vi "Find Inherited Test Methods in Test Case.vi"(8 "error in (no error)":errorcluster, 10 "Test Case Class Path":path, 11 "Test Finder In":refnum<class "Test Finder.lvclass">) -> (0 "error out":errorcluster, 2 "Test Methods Out":map{string, path}(c390), 3 "Test Finder Out":refnum<class "Test Finder.lvclass">)   [LabVIEW 2020, in "Test Finder.lvclass"]
uses:
  Test Finder.lvclass
  Test Case/LUnit Test Case.lvclass
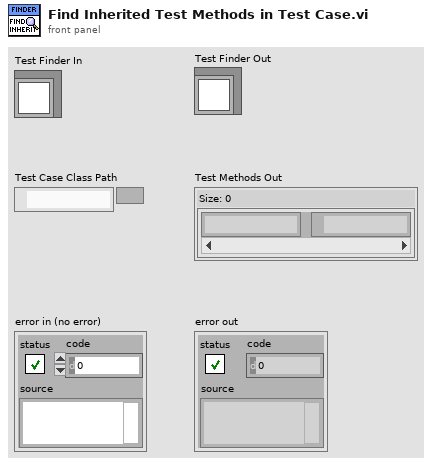
[diagram p1: front panel]
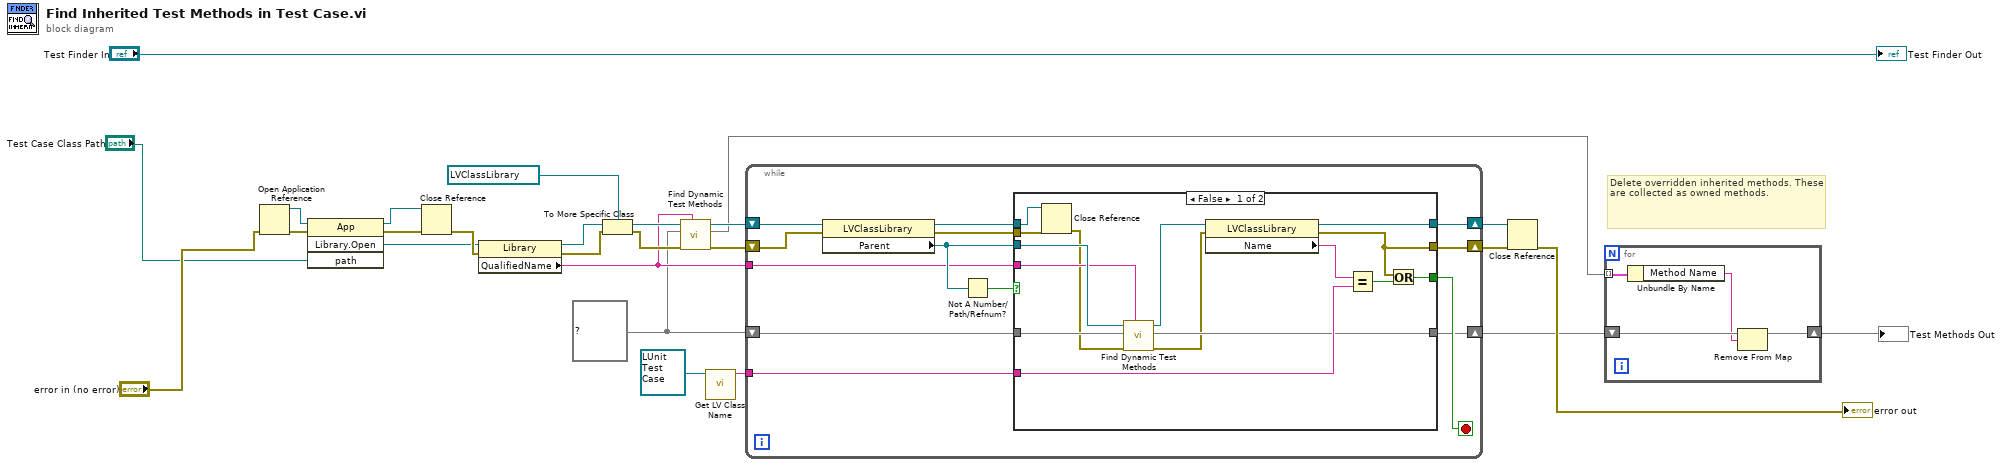
[diagram p0: block diagram]
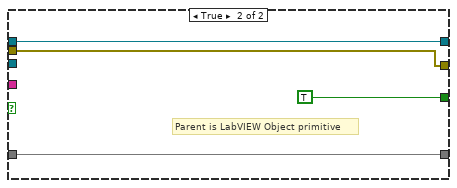
[diagram p2: hidden frame]
diagram:
  w4 = map{string, path} {} ("Test Methods In")
  # "Delete overridden inherited methods. These are collected as owned methods."
  n1 = Open Application Reference(8:"error in (no error)") -> (0:w25:errorcluster, 3:w26:refnum<vi>)  [unwired: 3 in]
  n2 = invoke on="Invoke Node" class="App" method="Library.Open"(reference=w26, error in=w25, "path"="Test Case Class Path") -> (reference out=w23:refnum<vi>, error out=w24:errorcluster, "Open Library"=w10:refnum<vi>)  [unwired: 1 in, 1 out]
  n3 = Close Reference(reference=w23, error in (no error)=w24) -> (error out=w14:errorcluster)
  n4 = property on="Property Node" class="Library"(reference=w10, error in=w14) -> (reference out=w15:refnum<vi>, error out=w13:errorcluster, "QualifiedName"=w5:string)
  n5 = To More Specific Class(target class=refnum<vi> refnum ("Library:Open"), reference=w15, error in=w13) -> (specific class reference=w9:refnum<vi>, error out=w7:errorcluster)
  n6 = call "Find Dynamic Test Methods.vi"("Test Case class name"=w5, "error in (no error)"=w7, "Test Methods In"=w4, "LVClassLibrary in"=w9) -> ("error out"=w6:errorcluster, "Test Methods Out"=w3:map{string, path}, "LVClassLibrary out"=w8:refnum<vi>)  [unwired: 5 in]
  n7 = call <vilib>:"Get LV Class Name.vi"("object"=refnum<class "LUnit Test Case.lvclass"> refnum ("Test Case in")) -> ("class name"=w18:string)  [unwired: 9 in, 1 out]
  n8 = while {
    shift-right: [w28] -> w2
    shift-left: w4 -> [w29]
    shift-right: [w38] -> w19
    shift-left: w8 -> [w31]
    shift-right: [w36] -> w21
    shift-left: w6 -> [w30]
    tunnel: w18 -> [w39]
    tunnel: w5 -> [w27]
    stop <- w37 stop-if-true
    n9 = property on="Property Node" class="LVClassLibrary"(reference=w31, error in=w30) -> (reference out=w33:refnum<vi>, error out=w32:errorcluster, "Parent"=w35:refnum<vi>)
    n10 = Not A Number/Path/Refnum?(number/path/refnum=w35) -> (NaN/Path/Refnum?=w34:bool)
    n11 = case shown="False" w34 {
      tunnel: w39 -> [w54 _]
      tunnel: [w53 w57] -> w38
      tunnel: [w52 TRUE] -> w37
      tunnel: [w51 w56] -> w36
      tunnel: w35 -> [w44 _]
      tunnel: w33 -> [w48 w57]
      tunnel: w32 -> [w47 w56]
      tunnel: w29 -> [w46 w55]
      tunnel: [w45 w55] -> w28
      tunnel: w27 -> [w42 _]
      frame False {
        n12 = Close Reference(reference=w48, error in (no error)=w47) -> (error out=w41:errorcluster)
        n13 = call "Find Dynamic Test Methods.vi"("Test Case class name"=w42, "error in (no error)"=w41, "Test Methods In"=w46, "LVClassLibrary in"=w44) -> ("error out"=w40:errorcluster, "Test Methods Out"=w45:map{string, path}, "LVClassLibrary out"=w43:refnum<vi>)  [unwired: 5 in]
        n14 = property on="Property Node" class="LVClassLibrary"(reference=w43, error in=w40) -> (reference out=w53:refnum<vi>, error out=w51:errorcluster, "Name"=w49:string)
        n15 = Equal?(x=w49, y=w54) -> (x = y?=w50:bool)
        n16 = Or(x=w51, y=w50) -> (x .or. y?=w52:bool)
      }
      frame True {
        # "Parent is LabVIEW Object primitive"
      }
    }
  }
  n17 = Close Reference(reference=w19, error in (no error)=w21) -> (error out=→"error out":errorcluster)
  n18 = for {
    tunnel: w3 -> [w60] mode=indexing
    shift-right: [w61] -> w1
    shift-left: w2 -> [w62]
    n19 = Unbundle By Name(w60) -> ("Method Name"=w59:string)
    n20 = Remove From Map(10:w59, 11:w62) -> (3:w61:map{string, path})  [unwired: 2 out]
  }
  "Test Methods Out" <- w1
  "Test Finder Out" <- "Test Finder In"
